vi "is_a_doc.vi"(7 "raise error if invalid? (False)":bool, 8 "error in (no error)":errorcluster, 11 "Doc in":refnum<class "Doc.lvclass">) -> (0 "error out":errorcluster, 3 "Doc out":refnum<class "Doc.lvclass">)   [LabVIEW 2020, in "toml_edit.lvlib" / "Doc.lvclass"]
uses:
  Doc.lvclass
  Doc.lvclass/Doc.ctl
panel:
  out "ref_is_valid?":bool
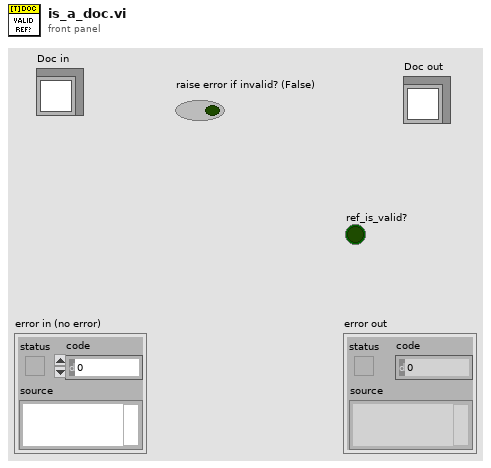
[diagram p1: front panel]
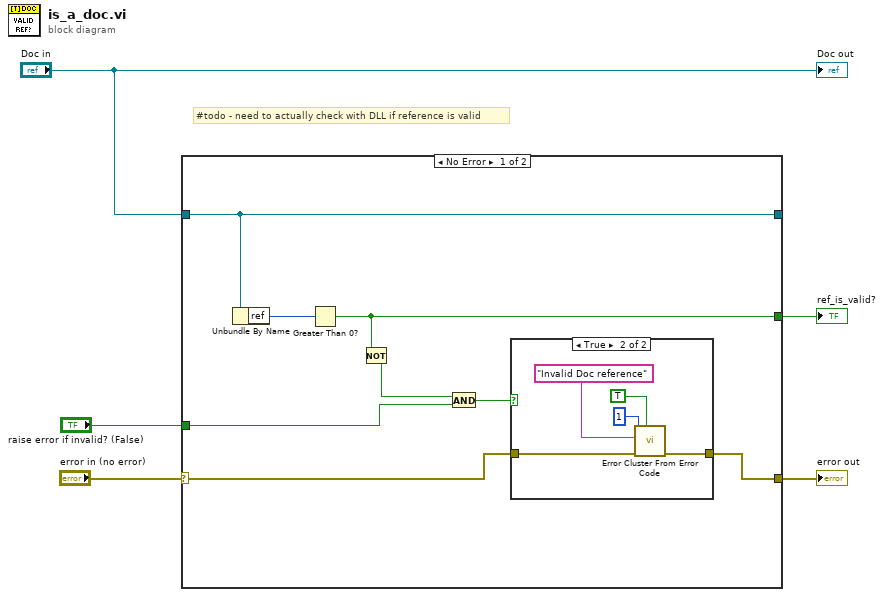
[diagram p0: block diagram]
diagram:
  # "#todo - need to actually check with DLL if reference is valid"
  n1 = case shown="No Error" "error in (no error)" {
    selector: "error in (no error)" -> [w9 w21]
    tunnel: [w8 w21] -> w4
    tunnel: [w13 w20] -> _
    tunnel: "Doc in" -> [w13 w20]
    tunnel: [w6 _] -> w3
    tunnel: "raise error if invalid? (False)" -> [w7 _]
    frame No Error {
      n2 = Unbundle By Name(w13) -> ("ref"=w12:u64)
      n3 = Greater Than 0?(x=w12) -> (x > 0?=w6:bool)
      n4 = Not(x=w6) -> (.not. x?=w10:bool)
      n5 = And(x=w10, y=w7) -> (x .and. y?=w11:bool)
      n6 = case shown="True" w11 {
        tunnel: [w14 w16] -> w8
        tunnel: w9 -> [w14 w15]
        frame False {
        }
        frame True {
          n7 = call <vilib>:"Error Cluster From Error Code.vi"("show call chain? (False)"=TRUE, "error in (no error)"=w15, "error message (\"\")"="Invalid Doc reference" ("error message (\"\")"), "error code (0)"=1) -> ("error out"=w16:errorcluster)  [unwired: 5 in]
        }
      }
    }
    frame Error {
    }
  }
  "error out" <- w4
  "ref_is_valid?" <- w3
  "Doc out" <- "Doc in"
